vi "select_elem_in_list (SubVI).vi"(11 "ListBox in":refnum<vi>) -> (3 "String":string)   [LabVIEW 2020]
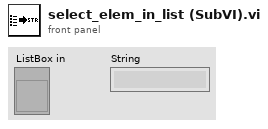
[diagram p1: front panel]
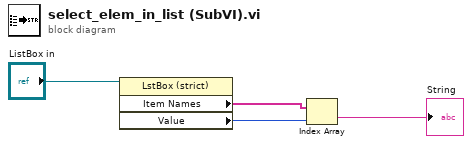
[diagram p0: block diagram]
diagram:
  n1 = property class="LstBox (strict)"(reference="ListBox in") -> ("Item Names"=w2:string[], "Value"=w3:i32)  [unwired: 1 in, 2 out]
  n2 = Index Array(array=w2, index=w3) -> (element=→"String":string)
